vi "TDMS Logger.vi"() -> ()   [LabVIEW 2010]
panel:
  out "시간 데이터":waveform(dbl)[](graph)
  out "파워 스펙트럼":waveform(dbl)[](graph)
  in  "UUT 시리얼 번호":string[](array[string])
  in  "테스트 수행자":string caption="Test Operator"
  in  "TDMS 파일 경로":path=path "D:/Exercises/LabVIEW Core 2/TDMS Logger/Test Data.tdms"
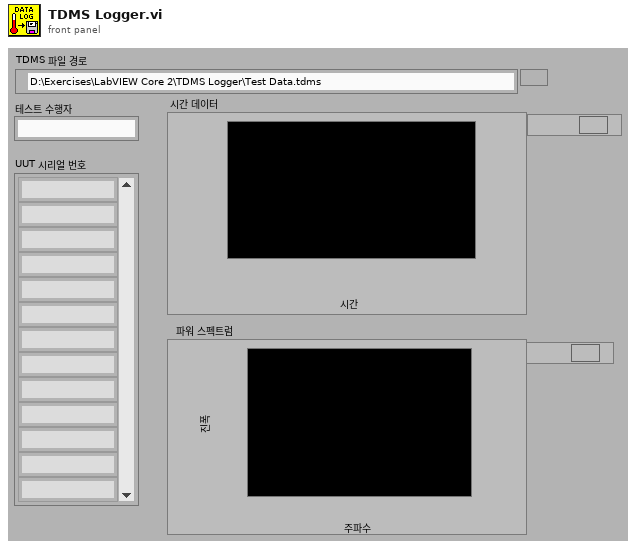
[diagram p1: front panel]
types:
  T1 = enum16{"open", "open or create", "create or replace", "create", "open (read-only)"}
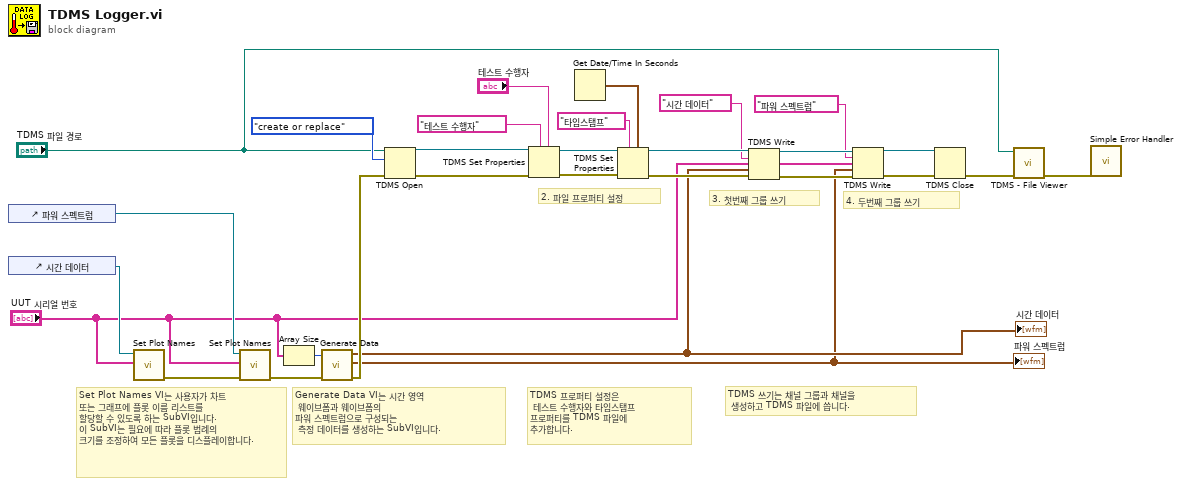
[diagram p0: block diagram]
diagram:
  # "4. 두번째 그룹 쓰기"
  # "3. 첫번째 그룹 쓰기"
  # "2. 파일 프로퍼티 설정"
  # "TDMS 프로퍼티 설정은 \n 테스트 수행자와 타임스탬프 \n프로퍼티를 TDMS 파일에 \n추가합니다."
  # "TDMS 쓰기는 채널 그룹과 채널을 \n 생성하고 TDMS 파일에 씁니다."
  # "Generate Data VI는 시간 영역\n 웨이브폼과 웨이브폼의 \n파워 스펙트럼으로 구성되는  \n 측정 데이터를 생성하는 SubVI입니다."
  # "Set Plot Names VI는 사용자가 차트 \n또는 그래프에 플롯 이름 리스트를 \n할당할 수 있도록 하는 SubVI입니다.\n이 SubVI는 필요에 따라 플롯 범례의 \n크기를 조정하여 모든 플롯을 디스플레이합니다."
  n1 = control-ref of="파워 스펙트럼"() -> (w30:refnum<vi>)
  n2 = control-ref of="시간 데이터"() -> (w26:refnum<vi>)
  n3 = call "Set Plot Names.vi"("플롯 이름"="UUT 시리얼 번호", "그래프 참조"=w26) -> ("에러 출력"=w29:errorcluster)  [unwired: 9 in]
  n4 = call "Set Plot Names.vi"("에러 입력(에러 없음)"=w29, "플롯 이름"="UUT 시리얼 번호", "그래프 참조"=w30) -> ("에러 출력"=w27:errorcluster)  [unwired: 8 in]
  n5 = Array Size(array="UUT 시리얼 번호") -> (size(s)=w28:i32)
  n6 = call "Generate Data.vi"("에러 입력"=w27, "채널 수"=w28) -> ("에러 출력"=w24:errorcluster, "파워 스펙트럼 데이터"=w9:waveform(dbl)[], "웨이브폼 차트"=w13:waveform(dbl)[])  [unwired: 7 in]
  "파워 스펙트럼" <- w9
  "시간 데이터" <- w13
  n7 = TDMS Open(8:w24, 10:T1."create or replace" ("operation (0:open)"), 11:"TDMS 파일 경로") -> (0:w18:errorcluster, 3:w23:refnum<k34>)  [unwired: 3 in]
  n8 = TDMS Set Properties(5:"테스트 수행자", 7:"테스트 수행자", 8:w18, 11:w23) -> (0:w22:errorcluster, 3:w21:refnum<k34>)  [unwired: 2 in, 2 out]
  n9 = Get Date/Time In Seconds() -> (seconds since 1Jan1904=w19:timestamp)
  n10 = TDMS Set Properties(5:w19, 7:"타임스탬프" ("Title"), 8:w22, 11:w21) -> (0:w16:errorcluster, 3:w17:refnum<k34>)  [unwired: 2 in, 2 out]
  n11 = TDMS Write(0:w17, 5:"시간 데이터" ("group name in (Untitled)"), 7:"UUT 시리얼 번호", 9:w13, 11:w16) -> (4:w12:refnum<k34>, 8:w8:string[], 15:w11:errorcluster)  [unwired: 1 in, 1 out]
  n12 = TDMS Write(0:w12, 5:"파워 스펙트럼" ("group name in (Untitled)"), 7:w8, 9:w9, 11:w11) -> (4:w7:refnum<k34>, 15:w6:errorcluster)  [unwired: 1 in, 2 out]
  n13 = TDMS Close(8:w6, 11:w7) -> (0:w5:errorcluster)  [unwired: 1 out]
  n14 = call <vilib>:"TDMS - File Viewer.vi"("error in (no error)"=w5, "file path"="TDMS 파일 경로") -> ("error out"=w3:errorcluster)  [unwired: 4 in, 1 out]
  n15 = call <vilib>:"Simple Error Handler.vi"("error in (no error)"=w3) -> ()  [unwired: 4 in, 5 out]
